vi "Configure Routing and Faulting Custom Device.vi"() -> ()   [LabVIEW 2019]
uses:
  SubVIs/Routing Channel Configuration.ctl
  NationalInstruments.VeriStand.SystemDefinitionAPI
  NI-SWITCH Examples.lvlib
  <vilib>/addons/VeriStand Custom Device Scripting APIs/Routing and Faulting/Scripting/Routing and Faulting Scripting.lvlib
panel:
  in  "Channel Configurations":T1[](array[typedef])=[{"Channel Name"="Window Up", "Initial State"="No Connections", "Description"="Window-Up Sensor State", "State Configurations"=[{"Name"="No Connections", "Description"="no connections", "Value"=-1.0, "Connection List"=[]}, {"Name"="Passthrough", "Description"="sensor connected", "Value"=1.0, "Connection List"=[{"Module Path"="Targets/Controller/Custom Devices/NI-SWITCH", "Source"="dut0", "Destination"="ch0"}]}, {"Name"="Short to Ground", "Description"="sensor faulted to ground", "Value"=2.0, "Connection List"=[{"Module Path"="Targets/Controller/Custom Devices/NI-SWITCH", "Source"="dut0", "Destination"="busa"}]}, {"Name"="Short to Power", "Description"="sensor faulted to power", "Value"=3.0, "Connection List"=[{"Module Path"="Targets/Controller/Custom Devices/NI-SWITCH", "Source"="dut0", "Destination"="busb"}]}, {"Name"="Open Circuit", "Description"="open circuit - not connected", "Value"=4.0, "Connection List"=[]}]}, {"Channel Name"="Window Down", "Initial State"="No Connections", "Description"="Window-Up Sensor State", "State Configurations"=[{"Name"="No Connections", "Description"="no connections", "Value"=-1.0, "Connection List"=[]}, {"Name"="Passthrough", "Description"="sensor connected", "Value"=1.0, "Connection List"=[{"Module Path"="Targets/Controller/Custom Devices/NI-SWITCH", "Source"="dut1", "Destination"="ch1"}]}, {"Name"="Short to Ground", "Description"="sensor faulted to ground", "Value"=2.0, "Connection List"=[{"Module Path"="Targets/Controller/Custom Devices/NI-SWITCH", "Source"="dut1", "Destination"="busa"}]}, {"Name"="Short to Power", "Description"="sensor faulted to power", "Value"=3.0, "Connection List"=[{"Module Path"="Targets/Controller/Custom Devices/NI-SWITCH", "Source"="dut1", "Destination"="busb"}]}, {"Name"="Open Circuit", "Description"="open circuit - not connected", "Value"=4.0, "Connection List"=[]}]}]
  in  "Output System Definition File":path=path "System Definition Files/System Definition with Routing and Faulting.nivssdf"
  in  "Input System Definition File (Preconfigured with an NI-SWITCH custom device)":path=path "System Definition Files/System Definition with NI-SWITCH.nivssdf"
  # "Overview: Demonstrates using the Routing and Faulting scripting API to configure the custom device. \n\nInstructions:\n1. Use one of the NI-SWITCH scripting examples (Configure NI-SWITCH Custom Device) to script one or more NI-SWITCH custom devices into a system definition file.\n2. Browse to the system definition created in step 1 to be used as the Input System Definition File.\n3. Browse to a path to save the system definition file as the output Output System Definition File.  This may be the same as the input file.\n4. For each routing channel you want to configure, use the Channel Configurations array to configure each channel's Name and Description.\n5. For each State, use the State Configurations array to set the State Name, Value, Description, and Connections List.\n6. For each Connection, set the Module path, Source endpoint, and Destination endpoint.\n7. After configurating each State, set the routing channel's Initial State (initial set of connections on deployment).\n8. Repeat steps 4-7 for each routing channel in your custom device.\n9. Run the VI and verify its results."
  # "System Definition Files"
  # "Routing and Faulting Custom Device Configuration"
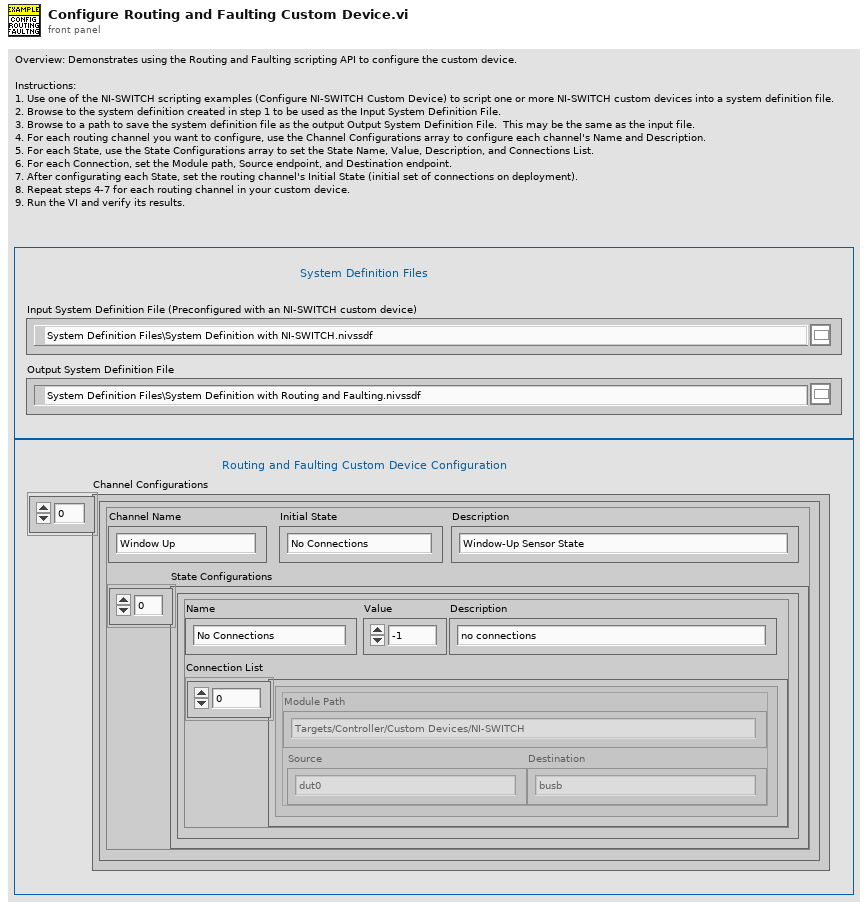
[diagram p1: front panel]
types:
  T1 = typedef "NI-SWITCH Examples.lvlib/Routing Channel Configuration.ctl" = cluster{"Channel Name":string, "Initial State":string, "Description":string, "State Configurations":cluster{"Name":string, "Description":string, "Value":dbl, "Connection List":cluster{"Module Path":string, "Source":string, "Destination":string}[]}[]}
  T2 = typedef "Custom Device API.lvlib/Custom Device Item Ref.ctl" = u64
  T3 = cluster{"Name":string, "Description":string, "Value":dbl, "Connection List":cluster{"Module Path":string, "Source":string, "Destination":string}[]}[]
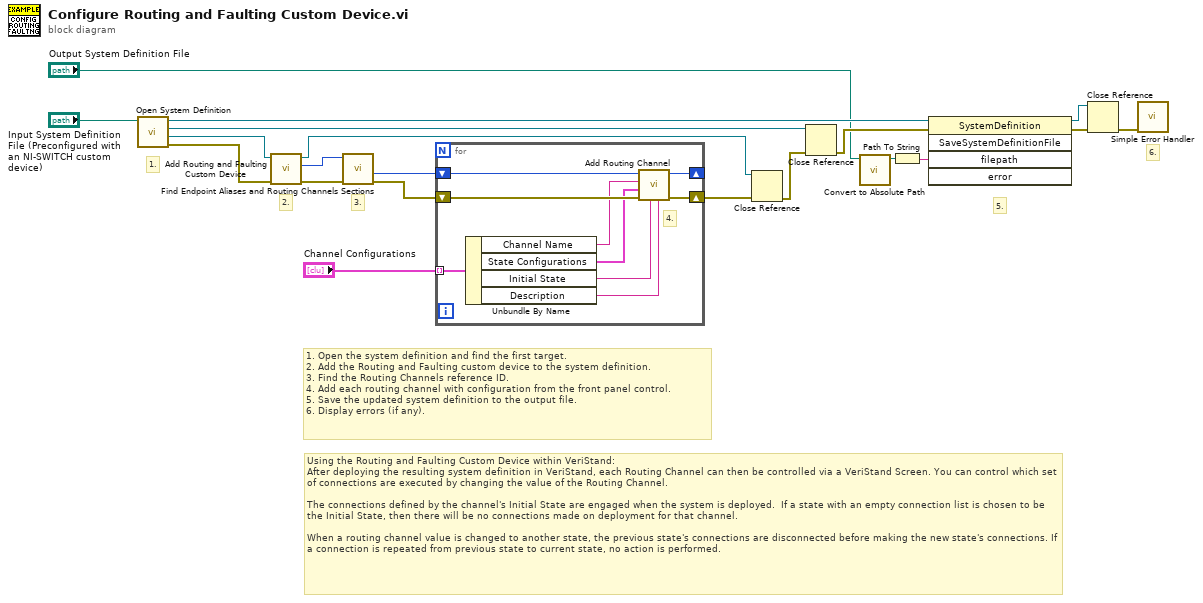
[diagram p0: block diagram]
diagram:
  # "Using the Routing and Faulting Custom Device within VeriStand:\nAfter deploying the resulting system definition in VeriStand, each Routing Channel can then be controlled via a VeriStand Screen. You can control which set of connections are executed by changing the value of the Routing Channel. \n\nThe connections defined by the channel's Initial State are engaged when the system is deployed.  If a state with an empty connection list is chosen to be the Initial State, then there will be no connections made on deployment for that channel.\n\nWhen a routing channel value is changed to another state, the previous state's connections are disconnected before making the new state's connections. If a connection is repeated from previous state to current state, no action is performed."
  # "3."
  # "2."
  # "5."
  # "6."
  # "8."
  # "1."
  # "1. Open the system definition and find the first target.\n2. Add the Routing and Faulting custom device to the system definition.\n3. Find the Routing Channels reference ID.\n4. Add each routing channel with configuration from the front panel control.\n5. Save the updated system definition to the output file.\n6. Display errors (if any)."
  n1 = call "Open System Definition.vi"("System Definition File"="Input System Definition File (Preconfigured with an NI-SWITCH custom device)") -> ("error out"=w2:errorcluster, "Target Refnum"=w10:refnum<k24>, "Root Refnum"=w16:refnum<k24>, "System Definition Refnum"=w20:refnum<k24>)  [unwired: 7 in]
  n2 = call <vilib>:"Add Routing and Faulting Custom Device.vi"("error in"=w2, "target in"=w10) -> ("error out"=w8:errorcluster, "routing and faulting custom device"=w9:T2, "target out"=w7:refnum<k24>)  [unwired: 7 in]
  n3 = call <vilib>:"Find Endpoint Aliases and Routing Channels Sections.vi"("error in"=w8, "routing and faulting custom device in"=w9) -> ("error out"=w6:errorcluster, "routing channels"=w5:T2)  [unwired: 6 in, 2 out]
  n4 = for {
    shift-right: [w27] -> w4
    shift-left: w6 -> [w29]
    shift-right: [w26] -> _
    shift-left: w5 -> [w28]
    tunnel: "Channel Configurations" -> [w25] mode=indexing
    # "4."
    n5 = Unbundle By Name(w25) -> ("Channel Name"=w23:string, "State Configurations"=w24:T3, "Initial State"=w22:string, "Description"=w21:string)
    n6 = call <vilib>:"Add Routing Channel.vi"("description"=w21, "initial state"=w22, "error in"=w29, "state configurations"=w24, "channel name"=w23, "routing channels in"=w28) -> ("error out"=w27:errorcluster, "routing channels out"=w26:T2)  [unwired: 3 in, 1 out]
  }
  n7 = Close Reference(reference=w7, error in (no error)=w4) -> (error out=w13:errorcluster)
  n8 = Close Reference(reference=w16, error in (no error)=w13) -> (error out=w15:errorcluster)
  n9 = call "Convert to Absolute Path.vi"("System Definition File"="Output System Definition File") -> ("Absolute Path"=w1:path)  [unwired: 10 in]
  n10 = Path To String(path=w1) -> (string=w19:string)
  n11 = invoke class="SystemDefinition" method="SaveSystemDefinitionFile"(reference=w20, error in=w15, "filepath"=w19) -> (reference out=w17:refnum<k24>, error out=w18:errorcluster)  [unwired: 2 in, 3 out]
  n12 = Close Reference(reference=w17, error in (no error)=w18) -> (error out=w12:errorcluster)
  n13 = call <vilib>:"Simple Error Handler.vi"("error in (no error)"=w12) -> ()  [unwired: 1 in, 8 out]
